vi "RT_RK4_translation (SubVI).vi"(8 "dt":dbl, 9 "dt*0.5":dbl, 10 "x(i)":dbl[](array[numeric]), 11 "acc":dbl) -> (3 "x(i+1)":dbl[](array[numeric]))   [LabVIEW 2017]
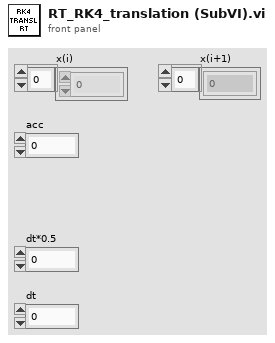
[diagram p1: front panel]
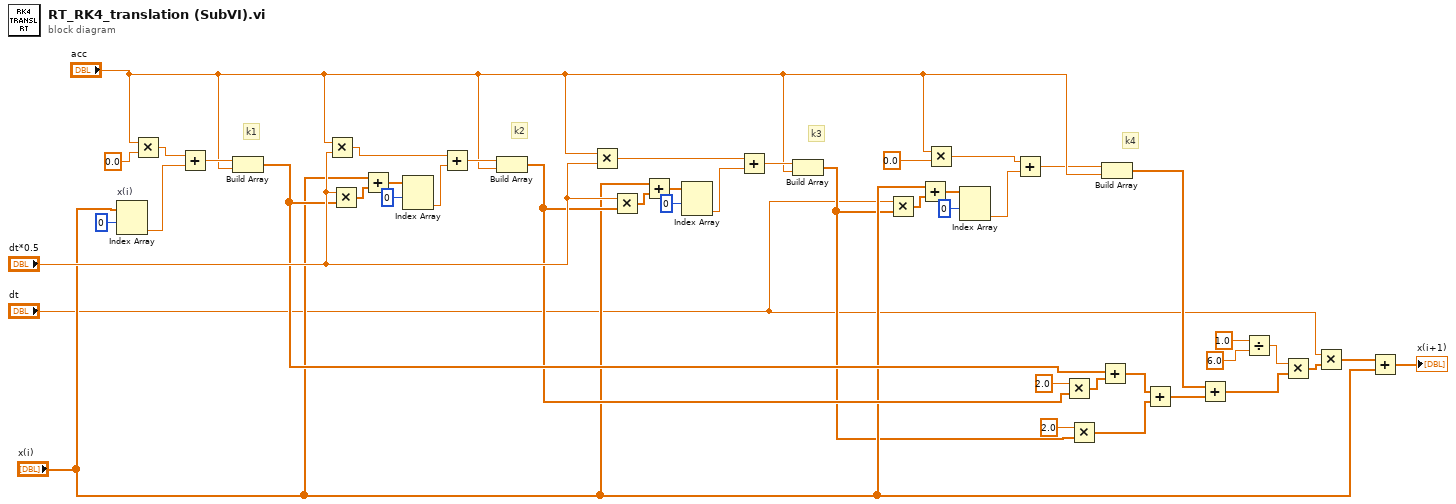
[diagram p0: block diagram]
diagram:
  # "k4"
  # "k3"
  # "k2"
  # "k1"
  n1 = Index Array "x(i)"(array="x(i)", index #1=0 ("index")) -> (element #2=w26:dbl)  [unwired: 1 in, 1 out]
  n2 = Multiply(x="acc", y=0.0) -> (x*y=w28:dbl)
  n3 = Add(x=w28, y=w26) -> (x+y=w19:dbl)
  n4 = Build Array(w19, "acc") -> (w17:dbl[])
  n5 = Multiply(x="acc", y="dt*0.5") -> (x*y=w30:dbl)
  n6 = Multiply(x="dt*0.5", y=w17) -> (x*y=w31:dbl[])
  n7 = Add(x="x(i)", y=w31) -> (x+y=w15:dbl[])
  n8 = Index Array(array=w15, index #1=0 ("index")) -> (element #2=w14:dbl)  [unwired: 1 in, 1 out]
  n9 = Add(x=w30, y=w14) -> (x+y=w23:dbl)
  n10 = Build Array(w23, "acc") -> (w13:dbl[])
  n11 = Multiply(x="acc", y="dt*0.5") -> (x*y=w33:dbl)
  n12 = Multiply(x="dt*0.5", y=w13) -> (x*y=w32:dbl[])
  n13 = Add(x="x(i)", y=w32) -> (x+y=w11:dbl[])
  n14 = Index Array(array=w11, index #1=0 ("index")) -> (element #2=w10:dbl)  [unwired: 1 in, 1 out]
  n15 = Add(x=w33, y=w10) -> (x+y=w22:dbl)
  n16 = Build Array(w22, "acc") -> (w3:dbl[])
  n17 = Multiply(x="dt", y=w3) -> (x*y=w6:dbl[])
  n18 = Add(x="x(i)", y=w6) -> (x+y=w8:dbl[])
  n19 = Multiply(x="acc", y=0.0) -> (x*y=w5:dbl)
  n20 = Index Array(array=w8, index #1=0 ("index")) -> (element #2=w9:dbl)  [unwired: 1 in, 1 out]
  n21 = Add(x=w5, y=w9) -> (x+y=w1:dbl)
  n22 = Multiply(x=2.0, y=w13) -> (x*y=w39:dbl[])
  n23 = Multiply(x=2.0, y=w3) -> (x*y=w43:dbl[])
  n24 = Add(x=w17, y=w39) -> (x+y=w41:dbl[])
  n25 = Build Array(w1, "acc") -> (w21:dbl[])
  n26 = Add(x=w41, y=w43) -> (x+y=w44:dbl[])
  n27 = Add(x=w21, y=w44) -> (x+y=w20:dbl[])
  n28 = Divide(x=1.0, y=6.0) -> (x/y=w38:dbl)
  n29 = Multiply(x=w38, y=w20) -> (x*y=w24:dbl[])
  n30 = Multiply(x="dt", y=w24) -> (x*y=w25:dbl[])
  n31 = Add(x=w25, y="x(i)") -> (x+y=→"x(i+1)":dbl[])
